vi "stream_only.vi"() -> ()   [LabVIEW 2025, in "LabJackEKG.lvlib"]
uses:
  LabJackEKG.lvlib
  Typedefs/AcqusitionConfig.ctl
  <vilib>/Analysis/NI_AALPro.lvlib
panel:
  out "Waveform Chart 2":i64(graph)
  in  "s":bool
  out "Waveform Graph":dbl[][](graph)
  in  "Sampling Frequency [Hz]":dbl=250.0
  out "stop":bool
  in  "milliseconds to wait":u32=100
  out "size(s)":i32
  out "Waveform Chart":cluster{dbl, dbl}(graph)
  in  "Number of Stickers":i64
  in  "Samping Window [s]":dbl
  out "error out":errorcluster
  in  "stop":bool
  in  "Acquisiton Config":T1 {"TC 2 Offset" format="%#_f"; "TC 2 Scale" format="%#_f"; "TC 1 Offset" format="%#_f"; "TC 1 Scale" format="%#_f"}
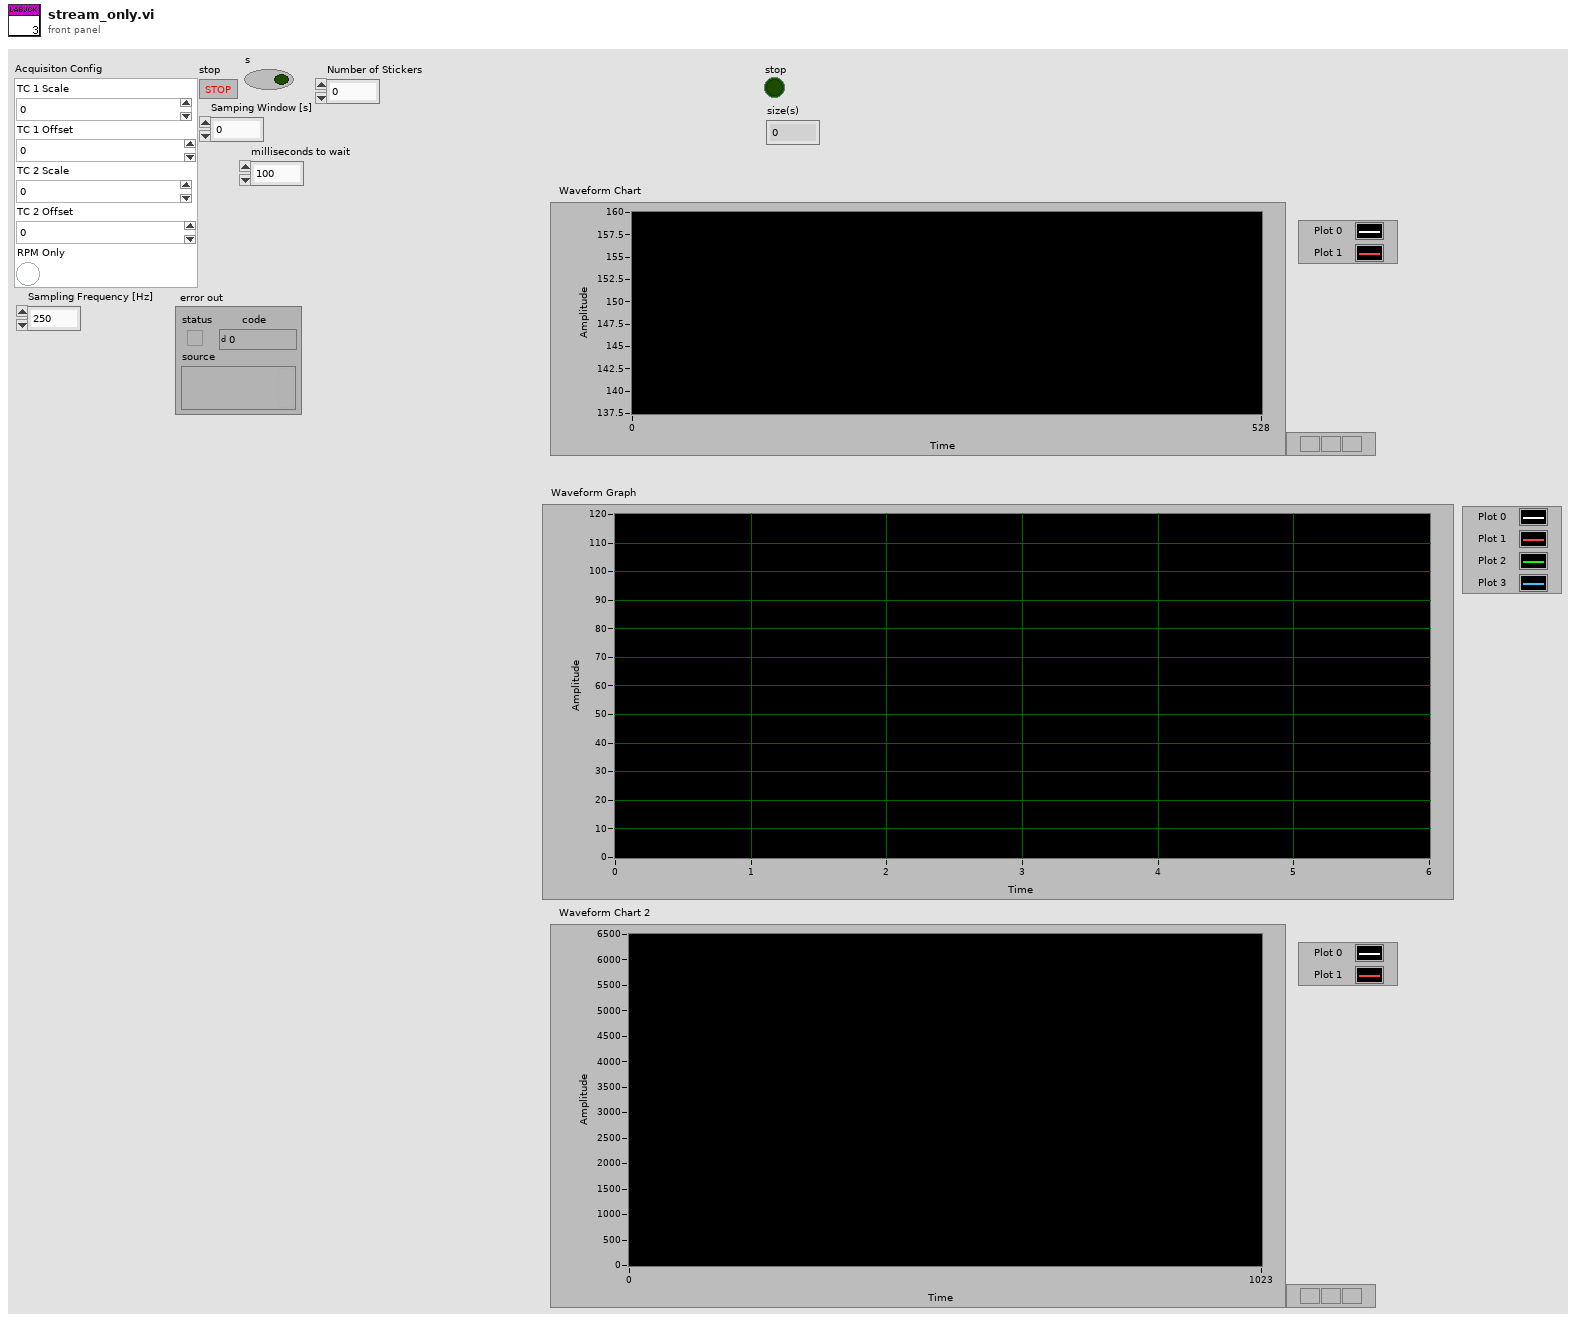
[diagram p1: front panel]
types:
  T1 = typedef "LabJackEKG.lvlib/AcqusitionConfig.ctl" = cluster{"TC 1 Scale":dbl, "TC 1 Offset":dbl, "TC 2 Scale":dbl, "TC 2 Offset":dbl, "RPM Only":bool}
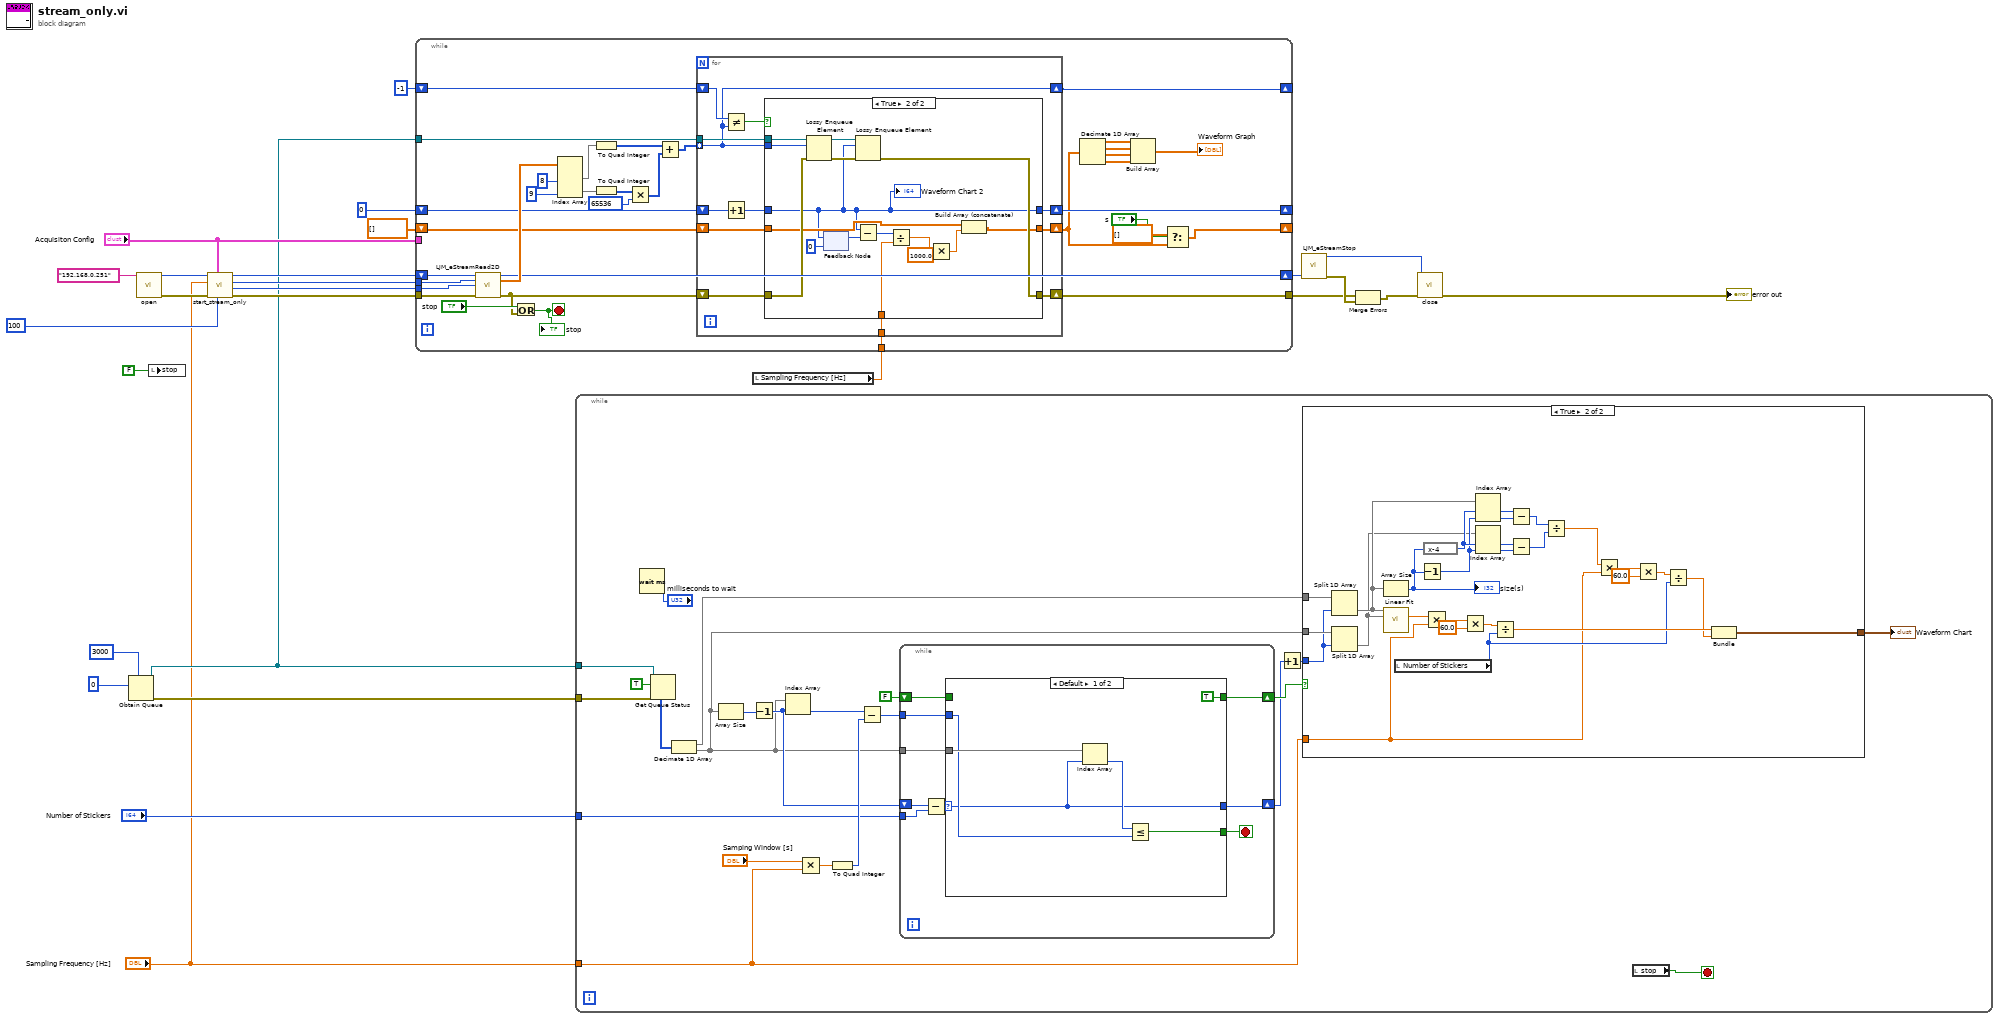
[diagram p0: block diagram]
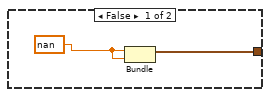
[diagram p2: hidden frame]
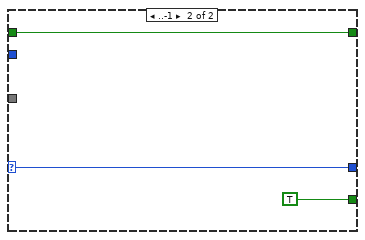
[diagram p3: hidden frame]
diagram:
  n1 = Obtain Queue(max queue size (-1, unlimited)=3000, element data type=i64 0) -> (queue out=w13:refnum<queue>, error out=w15:errorcluster)  [unwired: 3 in, 1 out]
  n2 = call "open.vi"("IP Address (LJM_idANY )"="192.168.0.251") -> ("error out"=w26:errorcluster, "Handle"=w25:i32)  [unwired: 8 in, 1 out]
  n3 = local write "stop"(FALSE ("x .or. y?")) -> ()
  n4 = call "start_stream_only.vi"("Period [ms]"=100, "AcqConfig"="Acquisiton Config", "error in (no error)"=w26, "Scan Rate (Hz)"="Sampling Frequency [Hz]", "Handle In"=w25) -> ("error out"=w24:errorcluster, "NumReadAddresses"=w20:i32, "ScansPerRead Out"=w21:i32, "Handle Out"=w23:i32)  [unwired: 3 in]
  n5 = while {
    tunnel: w13 -> [w48]
    tunnel: w15 -> [w47]
    tunnel: "Number of Stickers" -> [w40]
    tunnel: "Sampling Frequency [Hz]" -> [w29]
    stop <- w30 stop-if-true
    n6 = Wait (ms)(milliseconds to wait="milliseconds to wait") -> ()  [unwired: 1 out]
    n7 = Get Queue Status(queue=w48, return elements? (F)=TRUE, error in (no error)=w47) -> (elements=w46:i64[])  [unwired: 7 out]
    n8 = Decimate 1D Array(w46) -> (w35:i64[], w28:i64[])
    n9 = Array Size(array=w28) -> (size(s)=w37:i32)
    n10 = Decrement(x=w37) -> (x-1=w36:i32)
    n11 = Index Array(array=w28, index=w36) -> (element=w42:i64)
    n12 = Multiply(x="Samping Window [s]", y=w29) -> (x*y=w45:dbl)
    n13 = To Quad Integer(1:w45) -> (0:w43:i64)
    n14 = Subtract(x=w42, y=w43) -> (x-y=w41:i64)
    n15 = while {
      tunnel: w41 -> [w84]
      shift-right: [w81] -> w32
      shift-left: w36 -> [w78]
      tunnel: w40 -> [w86]
      tunnel: w28 -> [w80]
      shift-right: [w82] -> w34
      shift-left: FALSE -> [w79]
      stop <- w83 stop-if-true
      n16 = Subtract(x=w78, y=w86) -> (x-y=w85:i64)
      n17 = case shown="Default" w85 {
        selector: w85 -> [w88 w94]
        tunnel: w80 -> [w92 _]
        tunnel: w84 -> [w90 _]
        tunnel: [w89 TRUE] -> w83
        tunnel: [TRUE w93] -> w82
        tunnel: [w88 w94] -> w81
        tunnel: w79 -> [_ w93]
        frame Default {
          n18 = Index Array(array=w92, index=w88) -> (element=w91:i64)
          n19 = Less Or Equal?(x=w91, y=w90) -> (x <= y?=w89:bool)
        }
        frame ..-1 {
        }
      }
    }
    n20 = Increment(x=w32) -> (x+1=w31:i64)
    n21 = case shown="True" w34 {
      tunnel: w28 -> [_ w77]
      tunnel: w35 -> [_ w76]
      tunnel: w31 -> [_ w75]
      tunnel: w29 -> [_ w52]
      tunnel: [w50 w51] -> w27
      frame False {
        w49 = nan
        n22 = Bundle(w49, w49) -> (w50:cluster{dbl, dbl})  [unwired: 1 in]
      }
      frame True {
        n23 = Split 1D Array(array=w76, index=w75) -> (second subarray=w70:i64[])  [unwired: 1 out]
        n24 = Split 1D Array(array=w77, index=w75) -> (second subarray=w53:i64[])  [unwired: 1 out]
        n25 = Array Size(array=w70) -> (size(s)=w55:i32)
        "size(s)" <- w55
        n26 = call <vilib>:"Linear Fit.vi"("Y"=w70, "X"=w53) -> ("slope"=w61:dbl)  [unwired: 9 in, 4 out]
        n27 = local read "Number of Stickers"() -> (w57:i64)
        n28 = Decrement(x=w55) -> (x-1=w68:i32)
        n29 = expression code="x-4"(w55) -> (w69:i32)
        n30 = Multiply(x=w61, y=w52) -> (x*y=w74:dbl)
        n31 = Multiply(x=w74, y=60.0) -> (x*y=w73:dbl)
        n32 = Index Array(array=w70, index #1=w69, index #2=w68) -> (element #1=w65:i64, element #2=w64:i64)
        n33 = Index Array(array=w53, index #1=w69, index #2=w68) -> (element #1=w66:i64, element #2=w67:i64)
        n34 = Divide(x=w73, y=w57) -> (x/y=w71:dbl)
        n35 = Subtract(x=w65, y=w64) -> (x-y=w63:i64)
        n36 = Subtract(x=w66, y=w67) -> (x-y=w62:i64)
        n37 = Divide(x=w63, y=w62) -> (x/y=w54:dbl)
        n38 = Multiply(x=w54, y=w52) -> (x*y=w60:dbl)
        n39 = Multiply(x=w60, y=60.0) -> (x*y=w59:dbl)
        n40 = Divide(x=w59, y=w57) -> (x/y=w56:dbl)
        n41 = Bundle(w71, w56) -> (w51:cluster{dbl, dbl})  [unwired: 1 in]
      }
    }
    "Waveform Chart" <- w27
    n42 = local read "stop"() -> (w30:bool)
  }
  n43 = local read "Sampling Frequency [Hz]"() -> (w1:dbl)
  n44 = while {
    tunnel: w24 -> [w130]
    tunnel: [w119] -> w4
    tunnel: "Acquisiton Config" -> [_]
    tunnel: w21 -> [w128]
    tunnel: w20 -> [w129]
    shift-right: [w124] -> w8
    shift-left: w23 -> [w127]
    tunnel: w13 -> [w121]
    shift-right: [w114] -> _
    shift-left: i64 -1 -> [w115]
    shift-right: [w117] -> _
    shift-left: i64 0 -> [w118]
    shift-right: [w106] -> _
    shift-left: dbl[] [] -> [w108]
    tunnel: w1 -> [w102]
    stop <- w113 stop-if-true
    n45 = call <vilib>:"LJM_eStreamRead2D.vi"("Handle In"=w127, "ScansPerRead"=w128, "NumAddresses"=w129, "error in"=w130) -> ("Handle Out"=w124:i32, "aData Out"=w126:dbl[][], "error out"=w120:errorcluster)  [unwired: 7 in, 2 out]
    n46 = Or(x="stop", y=w120) -> (x .or. y?=w113:bool)
    "stop" <- w113
    n47 = Index Array(array=w126, index (col) #1=8 ("disabled index (col)"), index (col) #2=9 ("index (col)")) -> (element #1=w122:dbl[], element #2=w100:dbl[])  [unwired: 2 in]
    n48 = To Quad Integer(1:w122) -> (0:w116:i64[])
    n49 = To Quad Integer(1:w100) -> (0:w99:i64[])
    n50 = Multiply(x=w99, y=i64 65536 ("x")) -> (x*y=w96:i64[])
    n51 = Add(x=w116, y=w96) -> (x+y=w97:i64[])
    n52 = for {
      tunnel: w97 -> [w135] mode=indexing
      tunnel: w121 -> [w142]
      shift-right: [w141] -> w119
      shift-left: w120 -> [w140]
      shift-right: [w138] -> w117
      shift-left: w118 -> [w137]
      shift-right: [w135] -> w114
      shift-left: w115 -> [w136]
      shift-right: [w133] -> w103
      shift-left: w108 -> [w132]
      tunnel: w102 -> [w131]
      n53 = Not Equal?(x=w136, y=w135) -> (x != y?=w139:bool)
      n54 = Increment(x=w137) -> (x+1=w134:i64)
      n55 = case shown="True" w139 {
        tunnel: w142 -> [_ w161]
        tunnel: [w145 w157] -> w141
        tunnel: w140 -> [w145 w159]
        tunnel: w135 -> [_ w158]
        tunnel: [w144 w148] -> w138
        tunnel: w134 -> [w144 w148]
        tunnel: [w143 w150] -> w133
        tunnel: w132 -> [w143 w149]
        tunnel: w131 -> [_ w147]
        frame False {
        }
        frame True {
          n56 = Lossy Enqueue Element(queue=w161, element=w158, error in (no error)=w159) -> (queue out=w156:refnum<queue>, error out=w160:errorcluster)  [unwired: 2 out]
          n57 = feedback-in #1(w148) -> ()
          n58 = feedback #1(i64 0) -> (w155:i64)
          n59 = Lossy Enqueue Element(queue=w156, element=w148, error in (no error)=w160) -> (error out=w157:errorcluster)  [unwired: 3 out]
          n60 = Subtract(x=w148, y=w155) -> (x-y=w154:i64)
          n61 = Divide(x=w154, y=w147) -> (x/y=w152:dbl)
          n62 = Multiply(x=w152, y=1000.0) -> (x*y=w151:dbl)
          n63 = Build Array (concatenate)(w149, w151) -> (w150:dbl[])
          "Waveform Chart 2" <- w148
        }
      }
    }
    n64 = Decimate 1D Array(w103) -> (w109:dbl[], w110:dbl[], w111:dbl[], w112:dbl[])
    n65 = Build Array(w109, w110, w111, w112) -> (→"Waveform Graph":dbl[][])
    n66 = Select(t=dbl[] [], s="s", f=w103) -> (s? t:f=w106:dbl[])
  }
  n67 = call <vilib>:"LJM_eStreamStop.vi"("Handle In"=w8) -> ("Handle Out"=w7:i32, "error out"=w5:errorcluster)  [unwired: 13 in]
  n68 = Merge Errors(w4, w5) -> (w6:errorcluster)
  n69 = call "close.vi"("error in"=w6, "Handle"=w7) -> ("error out"=→"error out":errorcluster)  [unwired: 9 in]
